vi "ContextHelpEditor UI.vi"(6 "ComboBox Text":string, 7 "Executed on Frontpanel?":bool, 8 "error in (no error)":errorcluster, 11 "VI Ref":refnum<vi>) -> (0 "error out":errorcluster)   [LabVIEW 2017, in "ContextHelpEditor.lvlib"]
uses:
  ContextHelpEditor.lvlib
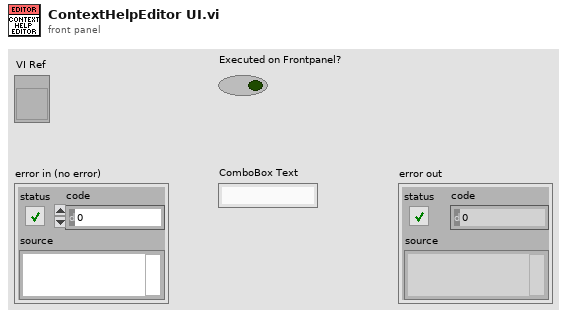
[diagram p1: front panel]
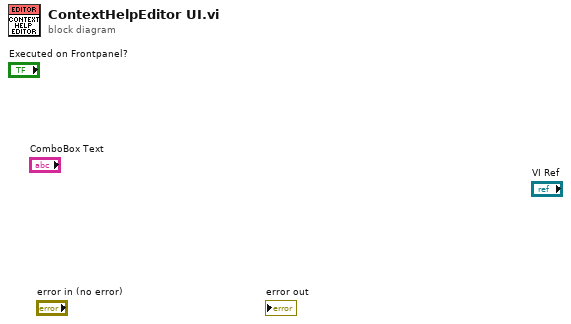
[diagram p0: block diagram]
diagram:
